vi "F to C main.vi"() -> ()   [LabVIEW 2012]
panel:
  in  "stop":bool
  in  "ON/OFF":bool
  out "Celcius":dbl(slide) scale=0.0..100.0
  in  "Farenheit":dbl(slide) scale=0.0..100.0
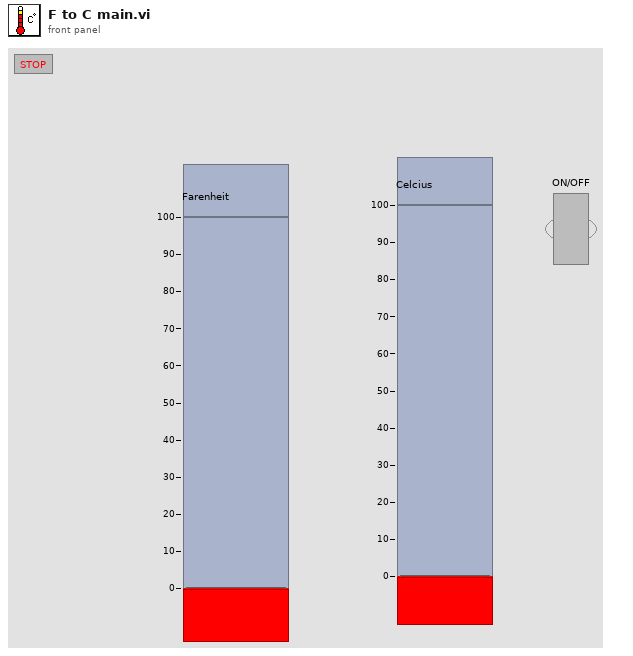
[diagram p1: front panel]
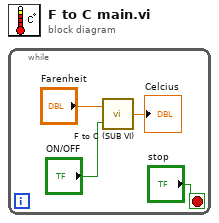
[diagram p0: block diagram]
diagram:
  n1 = while {
    stop <- "stop" stop-if-true
    n2 = call "F to C (SUB VI).vi"("Boolean"="ON/OFF", "Farenheit"="Farenheit") -> ("Celcius"=→"Celcius":dbl)
  }
